vi "Read Best Fit_.vi"(8 "Error In":errorcluster, 11 "Test in":refnum<class "Test.lvclass">) -> (0 "Error Out":errorcluster, 2 "Best Fit?":bool, 3 "Test out":refnum<class "Test.lvclass">)   [LabVIEW 2020, in "Test.lvclass"]
uses:
  Test.lvclass
  Test.lvclass/Test.ctl
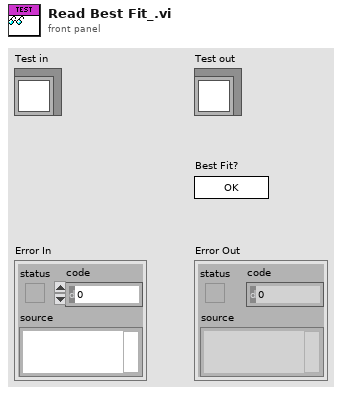
[diagram p1: front panel]
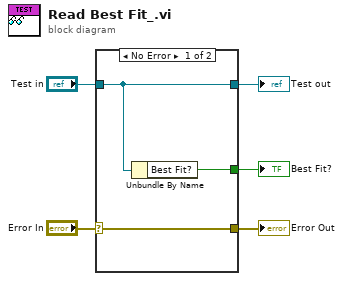
[diagram p0: block diagram]
diagram:
  n1 = case shown="No Error" "Error In" {
    selector: "Error In" -> [w8 w9]
    tunnel: [w8 w9] -> w4
    tunnel: [w7 w10] -> w2
    tunnel: "Test in" -> [w7 w10]
    tunnel: [w6 _] -> w1
    frame No Error {
      n2 = Unbundle By Name(w7) -> ("Best Fit?"=w6:bool)
    }
    frame Error {
    }
  }
  "Error Out" <- w4
  "Test out" <- w2
  "Best Fit?" <- w1
